vi "Move Tilt Stage Axis.vi"(0 "A":i32, 4 "Run A?":bool, 5 "B":i32=6, 6 "Run B?":bool, 7 "C":i32=4, 8 "Run C?":bool, 9 "A'":i32, 10 "Run A'?":bool, 11 "B'":i32=6, 15 "Run B'?":bool) -> ()   [LabVIEW 2016]
panel:
  out "error out 2":errorcluster caption="error out"
  out "error out":errorcluster
  out "Position of B'":i32
  out "Position of A'":i32
  out "Position of C":i32
  out "Position of B":i32
  out "Position of A":i32
  in  "stop":bool
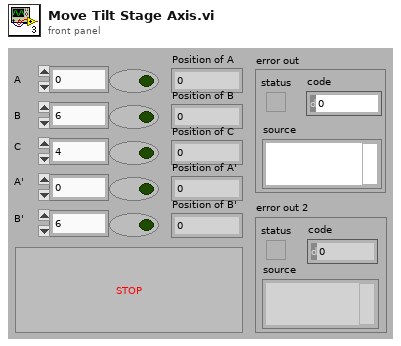
[diagram p1: front panel]
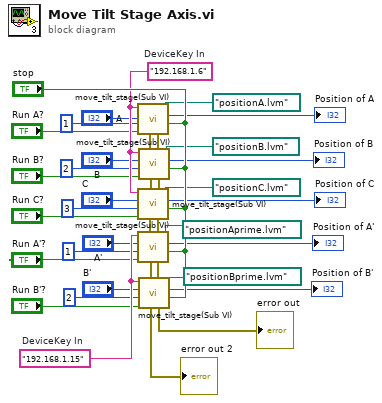
[diagram p0: block diagram]
diagram:
  w36 = "192.168.1.15"  # DeviceKey In
  w37 = "192.168.1.6"  # DeviceKey In
  n1 = call "move_tilt_stage(Sub VI).vi"("stop"="stop", "Filename"=path "positionA.lvm", "Boolean"="Run A?", "Motor Number"=1, "Relative Steps"="A", "DeviceKey In"=w37) -> ("Position Status"=→"Position of A":i32, "error out"=w2:errorcluster, "error out 2"=w3:errorcluster)  [unwired: 3 in]
  n2 = call "move_tilt_stage(Sub VI).vi"("stop"="stop", "Filename"=path "positionB.lvm", "error in (no error)"=w2, "error in (no error) 2"=w3, "Boolean"="Run B?", "Motor Number"=2, "Relative Steps"="B", "DeviceKey In"=w37) -> ("Position Status"=→"Position of B":i32, "error out"=w4:errorcluster, "error out 2"=w5:errorcluster)  [unwired: 1 in]
  n3 = call "move_tilt_stage(Sub VI).vi"("stop"="stop", "Filename"=path "positionC.lvm", "error in (no error)"=w4, "error in (no error) 2"=w5, "Boolean"="Run C?", "Motor Number"=3, "Relative Steps"="C", "DeviceKey In"=w37) -> ("Position Status"=→"Position of C":i32, "error out"=w7:errorcluster, "error out 2"=w6:errorcluster)  [unwired: 1 in]
  n4 = call "move_tilt_stage(Sub VI).vi"("stop"="stop", "Filename"=path "positionAprime.lvm", "error in (no error)"=w7, "error in (no error) 2"=w6, "Boolean"="Run A'?", "Motor Number"=1, "Relative Steps"="A'", "DeviceKey In"=w36) -> ("Position Status"=→"Position of A'":i32, "error out"=w8:errorcluster, "error out 2"=w9:errorcluster)  [unwired: 1 in]
  n5 = call "move_tilt_stage(Sub VI).vi"("stop"="stop", "Filename"=path "positionBprime.lvm", "error in (no error)"=w8, "error in (no error) 2"=w9, "Boolean"="Run B'?", "Motor Number"=2, "Relative Steps"="B'", "DeviceKey In"=w36) -> ("Position Status"=→"Position of B'":i32, "error out"=→"error out":errorcluster, "error out 2"=→"error out 2":errorcluster)  [unwired: 1 in]
